vi "GetExample.vi"(9 "# Devices":enum32{"Page 1", "Page 2", "Page 3"}(ring), 10 "Listbox":i32, 11 "ListBox in":refnum<vi>) -> (1 "image":picture, 2 "description":string, 3 "name":string, 4 "Python":string)   [LabVIEW 2016]
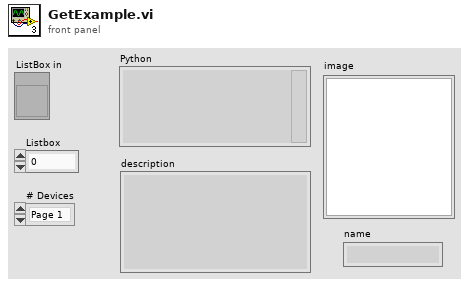
[diagram p1: front panel]
types:
  T1 = typedef "imagedata.ctl" = cluster{"image type":i32, "image depth":i32, "image":u8[], "mask":u8[], "colors":u32[], "Rectangle":cluster{"left":i16, "top":i16, "right":i16, "bottom":i16}}
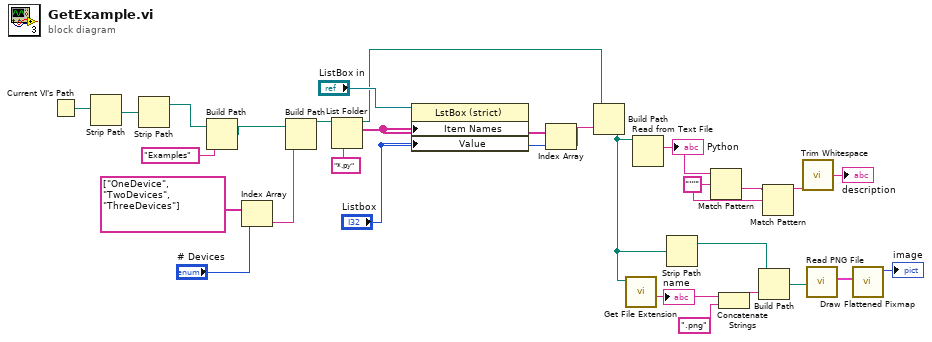
[diagram p0: block diagram]
diagram:
  w11 = "'''" ("regular expression")
  n1 = Current VI's Path() -> (path=w21:path)
  n2 = Strip Path(path=w21) -> (stripped path=w17:path)  [unwired: 1 out]
  n3 = Strip Path(path=w17) -> (stripped path=w16:path)  [unwired: 1 out]
  n4 = Build Path(base path=w16, name or relative path="Examples") -> (appended path=w26:path)
  n5 = Index Array(array=string[] ["OneDevice", "TwoDevices", "ThreeDevices"], index="# Devices") -> (element=w28:string)
  n6 = Build Path(base path=w26, name or relative path=w28) -> (appended path=w27:path)
  n7 = List Folder(path=w27, pattern="*.py") -> (path out=w14:path, filenames=w19:string[])  [unwired: 2 in, 2 out]
  n8 = property on="Property Node" class="LstBox (strict)"(reference="ListBox in", "Item Names"=w19, "Value"="Listbox") -> ()  [unwired: 1 in, 2 out]
  n9 = Index Array(array=w19, index="Listbox") -> (element=w15:string)
  n10 = Build Path(base path=w14, name or relative path=w15) -> (appended path=w6:path)
  n11 = call <vilib>:"Get File Extension.vi"("file"=w6) -> ("filename without extension"=w8:string)  [unwired: 6 in, 4 out]
  "name" <- w8
  n12 = Read from Text File(file (use dialog)=w6) -> (text=w13:string)  [unwired: 3 in, 3 out]
  "Python" <- w13
  n13 = Strip Path(path=w6) -> (stripped path=w4:path)  [unwired: 1 out]
  n14 = Match Pattern(string=w13, regular expression=w11) -> (after substring=w12:string)  [unwired: 1 in, 3 out]
  n15 = Concatenate Strings(w8, ".png" ("string")) -> (w5:string)
  n16 = Build Path(base path=w4, name or relative path=w5) -> (appended path=w3:path)
  n17 = Match Pattern(string=w12, regular expression=w11) -> (before substring=w10:string)  [unwired: 1 in, 3 out]
  n18 = call <vilib>:"Trim Whitespace.vi"("string"=w10) -> ("trimmed string"=→"description":string)  [unwired: 1 in]
  n19 = call <vilib>:"Read PNG File.vi"("path to PNG file"=w3) -> ("image data"=w2:T1)  [unwired: 8 in, 2 out]
  n20 = call <vilib>:"Draw Flattened Pixmap.vi"("image data"=w2) -> ("new picture"=→"image":picture)  [unwired: 8 in]
